vi "Write State change time.vi"(8 "error in (no error)":errorcluster, 10 "State change time":timestamp, 11 "BiStableShutter in":refnum<class "BiStableShutter.lvclass">) -> (0 "error out":errorcluster, 3 "BiStableShutter out":refnum<class "BiStableShutter.lvclass">)   [LabVIEW 2016, in "BiStableShutter.lvclass"]
uses:
  BiStableShutter.lvclass
  BiStableShutter.lvclass/BiStableShutter.ctl
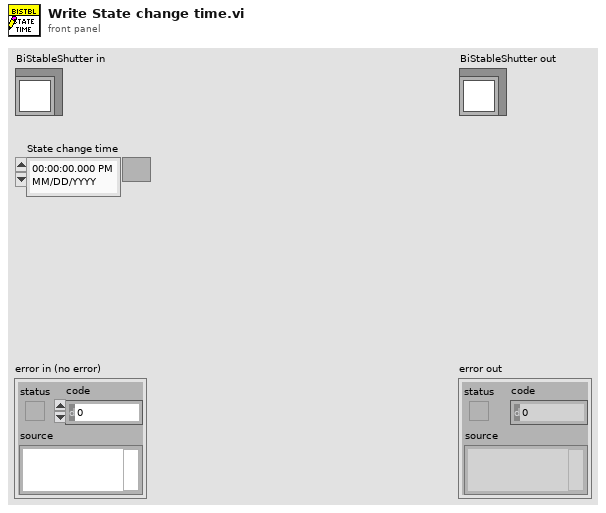
[diagram p1: front panel]
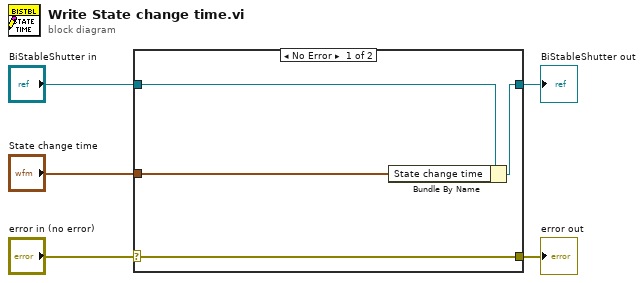
[diagram p0: block diagram]
diagram:
  n1 = case shown="No Error" "error in (no error)" {
    selector: "error in (no error)" -> [w9 w10]
    tunnel: [w9 w10] -> w4
    tunnel: [w7 w11] -> w2
    tunnel: "BiStableShutter in" -> [w8 w11]
    tunnel: "State change time" -> [w6 _]
    frame No Error {
      n2 = Bundle By Name(cluster=w8, "State change time"=w6) -> (w7:refnum<class "BiStableShutter.lvclass">)
    }
    frame Error {
    }
  }
  "error out" <- w4
  "BiStableShutter out" <- w2
